vi "Mod_OFDM_Rx.vi"(0 "input complex waveform":T2={"t0"=0.0, "dt"=1.0, "Y"=[]} {"Y" format="%.3f"; "dt" format="%^.2e"; "t0" format="%.4f"}, 1 "Complex Symbols w/ Cyclic prefix":cdb[](array[numeric]), 2 "BitsTransmitted":i8[](array[numeric]), 5 "Parameters per Ofdm Symbol":T3 {"Data Source"."Data Source"."Register Initial State" format="%08x"}, 7 "matched filter coefficients":dbl[](array[numeric]) format="%^.2e", 9 "Pulse Shaping":T4={"System Filter"={"TX Filter"=enum."Root Raised Cos", "Alpha"=0.5, "filter length"=8}, "Modulation system parameters"={"samples per symbol (16)"=16}, "symbol rate (Hz)"=1.0} {"symbol rate (Hz)" min=1.0 step=1.0 format="%.2p"; "Modulation system parameters"."samples per symbol (16)" step=2; "System Filter"."Alpha" min=0.0 max=1.0 step=0.05 format="%.2f"}, 11 "error in (no error)":errorcluster, 13 "reset? (T)":bool=TRUE) -> (3 "complex waveform Down Sampled":T2 {"Y" format="%.3f"; "dt" format="%^.2e"; "t0" format="%.4f"}, 4 "o/p":T1, 15 "error out":errorcluster)   [LabVIEW 2010]
doc: "This VI implements a generic OFDM receiver"
uses:
  <vilib>/addons/Modulation/Analog/controls/Complex Data Waveform.ctl
  Controls(Type_DEf)/Configure Pulse Shaping.ctl
  Controls(Type_DEf)/Parameters per Ofdm Symbol.ctl
panel:
  out "Offset":i32
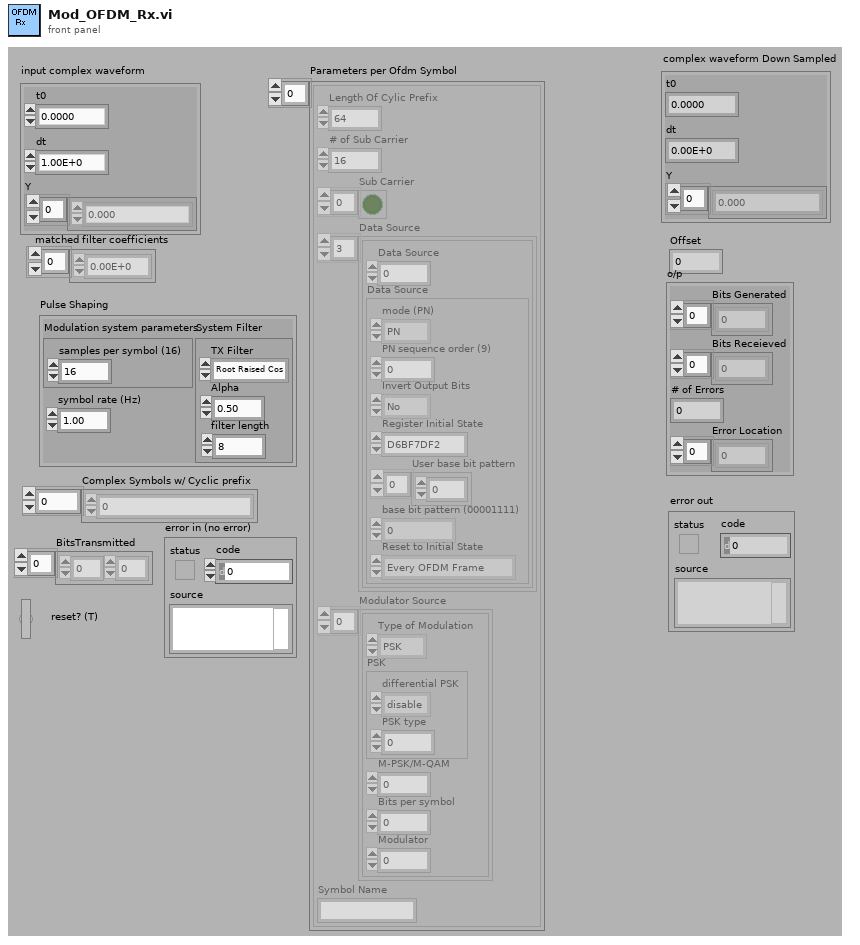
[diagram p1: front panel]
types:
  T1 = cluster{"Bits Generated":i8[], "Bits Receieved":i8[], "# of Errors":i32, "Error Location":i32[]}
  T2 = typedef "Complex Data Waveform.ctl" = cluster{"t0":dbl, "dt":dbl, "Y":cdb[]}
  T3 = typedef "Parameters per Ofdm Symbol.ctl" = cluster{"Length Of Cylic Prefix":i32, "# of Sub Carrier":i32, "Sub Carrier":bool[], "Data Source":cluster{"Data Source":u16, "Data Source":cluster{"mode (PN)":enum16{"PN", "pattern", "user"}, "PN sequence order (9)":i32, "Invert Output Bits":enum16{"No", "Yes"}, "Register Initial State":u32, "User base bit pattern":i8[], "base bit pattern (00001111)":enum16{"0", "1", "01", "0011", "00001111"}, "Reset to Initial State":enum16{"Every OFDM Frame", "Every OFDM Symbol", "Every Sub Carrier"}}}[], "Modulator Source":cluster{"Type of Modulation":enum16{"PSK", "QAM"}, "PSK":cluster{"differential PSK":enum16{"disable", "enable"}, "PSK type":u16}, "M-PSK/M-QAM":i32, "Bits per symbol":i32, "Modulator":u16}[], "Symbol Name":string}[]
  T4 = typedef "Configure Pulse Shaping.ctl" = cluster{"System Filter":cluster{"TX Filter":enum16{"none", "Raised Cosine", "Root Raised Cos"}, "Alpha":dbl, "filter length":i32}, "Modulation system parameters":cluster{"samples per symbol (16)":u32}, "symbol rate (Hz)":dbl}
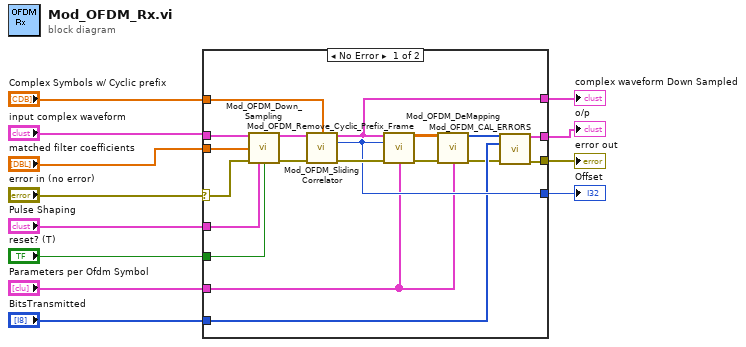
[diagram p0: block diagram]
diagram:
  n1 = case shown="No Error" "error in (no error)" {
    selector: "error in (no error)" -> [w18 w32]
    tunnel: [w28 _] -> w12
    tunnel: [w27 _] -> w11
    tunnel: "input complex waveform" -> [w24 _]
    tunnel: "matched filter coefficients" -> [w23 _]
    tunnel: "Complex Symbols w/ Cyclic prefix" -> [w22 _]
    tunnel: "BitsTransmitted" -> [w16 _]
    tunnel: [w13 w32] -> w6
    tunnel: "Parameters per Ofdm Symbol" -> [w21 _]
    tunnel: "Pulse Shaping" -> [w20 _]
    tunnel: "reset? (T)" -> [w19 _]
    tunnel: [w14 _] -> w1
    frame No Error {
      n2 = call "Mod_OFDM_Down_Sampling.vi"("input complex waveform"=w24, "matched filter coefficients"=w23, "error in (no error)"=w18, "Pulse Shaping"=w20, "reset? (T)"=w19) -> ("output complex waveform"=w25:T2, "error out"=w30:errorcluster)  [unwired: 9 in]
      n3 = call "Mod_OFDM_Sliding Correlator.vi"("complex waveform Down Sampled"=w25, "Complex Signal Generated"=w22, "error in (no error)"=w30) -> ("complex waveform Down Sampled"=w27:T2, "Offset"=w28:i32, "error out"=w29:errorcluster)  [unwired: 10 in]
      n4 = call "Mod_OFDM_Remove_Cyclic_Prefix_Frame.vi"("output complex\nwaveform"=w27, "Offset"=w28, "error in (no error)"=w29, "Parameters per Ofdm Symbol"=w21) -> ("FFT {X}"=w31:cdb[][], "error out"=w26:errorcluster)  [unwired: 9 in, 1 out]
      n5 = call "Mod_OFDM_DeMapping.vi"("FFT {X}"=w31, "error in (no error)"=w26, "Parameters per Ofdm Symbol"=w21) -> ("Bits Out"=w17:i8[], "error out"=w15:errorcluster)  [unwired: 11 in]
      n6 = call "Mod_OFDM_CAL_ERRORS.vi"("Bits Received"=w17, "BitsTransmitted"=w16, "error in (no error)"=w15) -> ("O/P"=w14:T1, "error out"=w13:errorcluster)  [unwired: 11 in]
    }
    frame Error {
    }
  }
  "error out" <- w6
  "complex waveform Down Sampled" <- w11
  "Offset" <- w12
  "o/p" <- w1
